vi "Raft_wars_Ver8.vi"() -> ()   [LabVIEW 2026]
panel:
  in  "Play Again":bool
  out "Computer Board":dbl[][](array[numeric])
  out "Player  Board":dbl[][](array[numeric])
  in  "Player Ship Inputs":T1(array[cluster]) {"Y-Coordinate" min=0 max=7; "X-Coordinate" min=0 max=7}
  in  "Emergency Stop":bool
  out "Game Status":string
  out "Ships Placed":dbl
  out "Losses":dbl
  out "Computer Hits":dbl
  out "Wins":dbl
  out "Player Hits":dbl
  in  "Attack":bool
  in  "Place Ship":bool
  in  "Attack Y":dbl
  in  "Attack X":dbl
  in  "Ship Y":dbl
  in  "Ship X":dbl
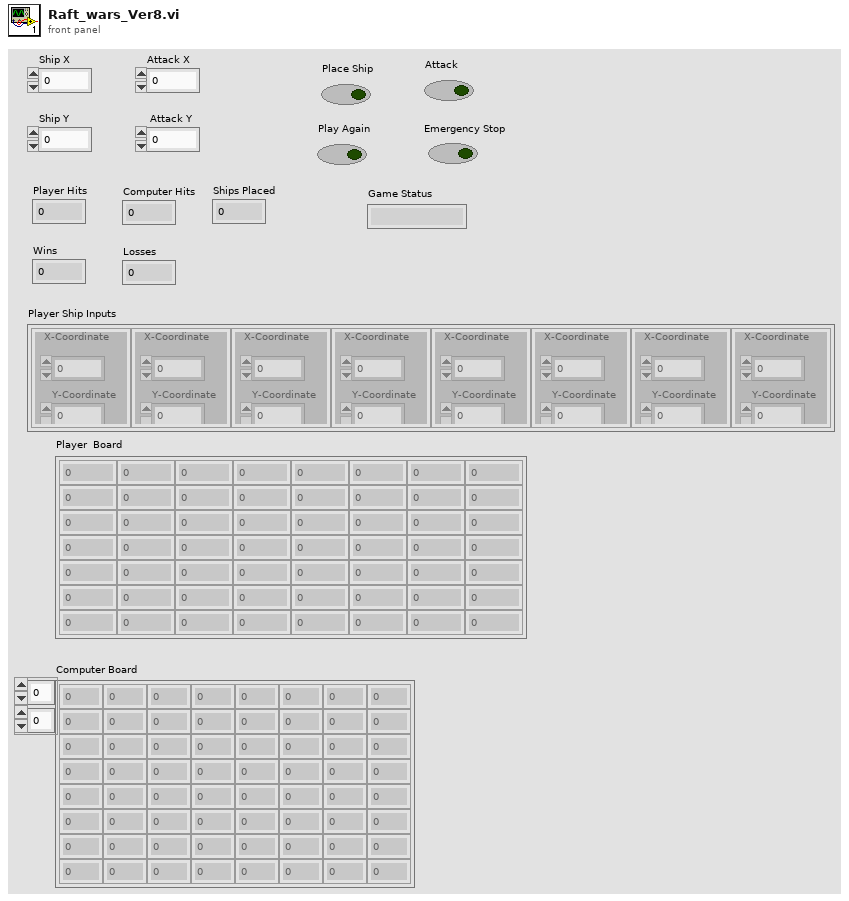
[diagram p1: front panel]
types:
  T1 = cluster{"X-Coordinate":i32, "Y-Coordinate":i32}[]
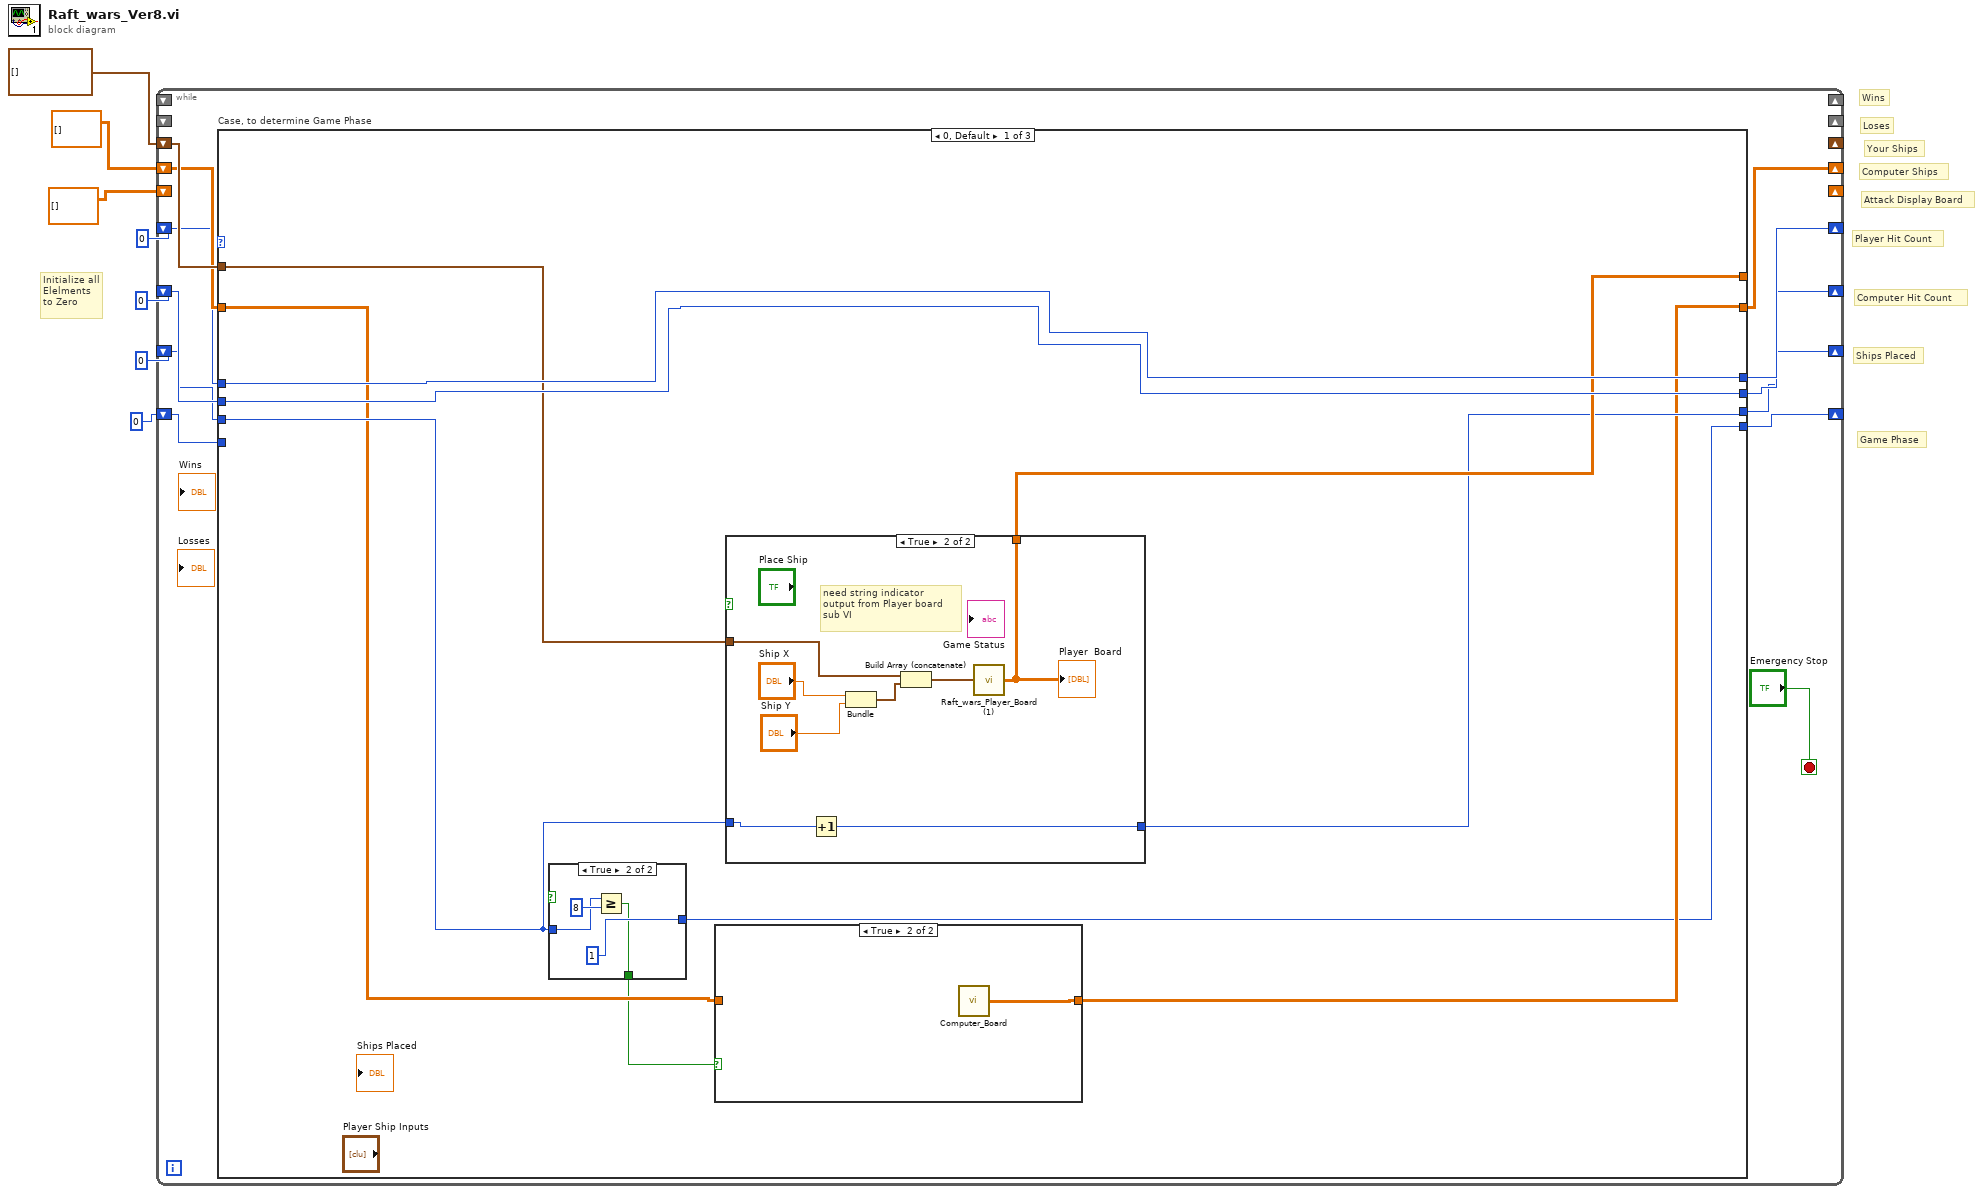
[diagram p0: block diagram]
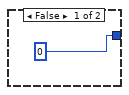
[diagram p3: hidden frame]
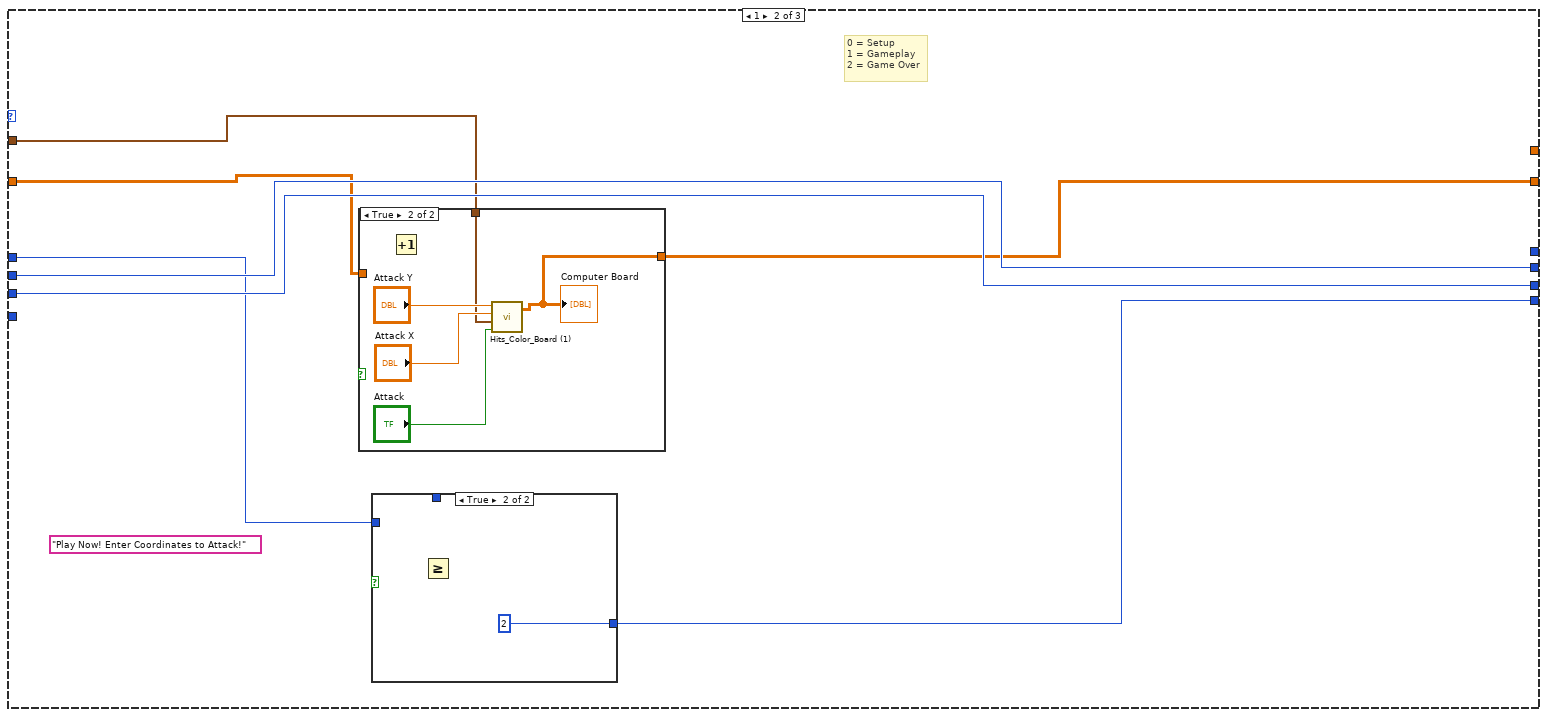
[diagram p5: hidden frame]
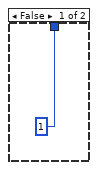
[diagram p6: hidden frame]
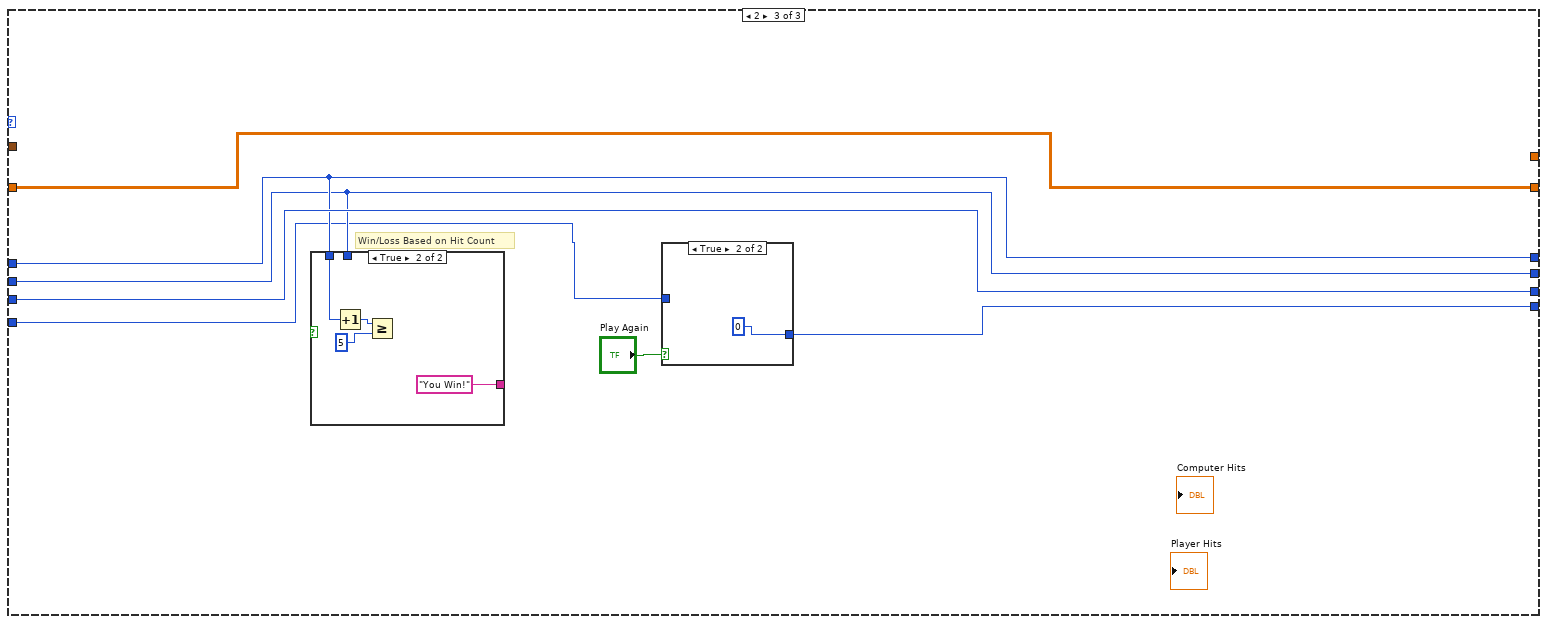
[diagram p8: hidden frame]
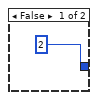
[diagram p9: hidden frame]
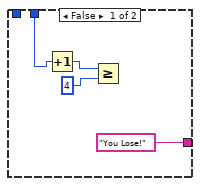
[diagram p10: hidden frame]
diagram:
  # "Loses"
  # "Wins"
  # "Attack Display Board"
  # "Initialize all\nElelments\nto Zero"
  # "Ships Placed"
  # "Your Ships"
  # "Computer Ships"
  # "Player Hit Count"
  # "Computer Hit Count"
  # "Game Phase"
  n1 = while {
    shift-right: _ -> [_]
    shift-left: cluster{i32, i32}[] [] -> [w18]
    shift-right: [w9] -> _
    shift-left: dbl[][] [] ("Array") -> [w17]
    shift-right: [w13] -> _
    shift-left: 0 -> [w16]
    shift-right: [w12] -> _
    shift-left: 0 -> [w15]
    shift-right: [w11] -> _
    shift-left: 0 -> [w14]
    shift-right: [w10] -> _
    shift-left: 0 -> [w8]
    shift-right: _ -> [_]
    shift-left: dbl[][] [] ("Array") -> [_]
    shift-right: _ -> [_]
    shift-left: _ -> [_]
    shift-right: _ -> [_]
    shift-left: _ -> [_]
    stop <- "Emergency Stop" stop-if-true
    n2 = case "Case, to determine Game Phase" shown="0, Default" {
      selector: _ -> [_ _ _]
      tunnel: w18 -> [w27 w46 _]
      tunnel: [w25 _ _] -> _
      tunnel: w17 -> [w21 w48 w66]
      tunnel: [w23 w49 w66] -> w9
      tunnel: w16 -> [w29 w47 w64]
      tunnel: w15 -> [w28 w51 w63]
      tunnel: w14 -> [w26 w52 w65]
      tunnel: [w29 _ w64] -> w13
      tunnel: [w28 w51 w63] -> w12
      tunnel: [w24 w52 w65] -> w11
      tunnel: [w22 w50 w62] -> w10
      tunnel: w8 -> [_ _ w60]
      frame 0, Default {
        n3 = case shown="True" {
          selector: _ -> [_ _]
          tunnel: w26 -> [_ w35]
          tunnel: [0 1] -> w22
          tunnel: [_ w33] -> w20
          frame False {
          }
          frame True {
            n4 = Greater Or Equal?(x=w35, y=8) -> (x >= y?=w33:bool)
          }
        }
        n5 = case shown="True" w20 {
          tunnel: w21 -> [w30 _]
          tunnel: [w30 w31] -> w23
          frame False {
          }
          frame True {
            n6 = call "Computer_Board.vi"() -> ("Array"=w31:dbl[][])
          }
        }
        n7 = case shown="True" {
          selector: _ -> [_ _]
          tunnel: w27 -> [_ w41]
          tunnel: w26 -> [w37 w39]
          tunnel: [_ w40] -> w25
          tunnel: [w37 w38] -> w24
          frame False {
          }
          frame True {
            # "need string indicator\noutput from Player board \nsub VI"
            n8 = Increment(x=w39) -> (x+1=w38:i32)
            n9 = Bundle("Ship X"="Ship X", "Ship Y"="Ship Y") -> (w43:cluster{"Ship X":dbl, "Ship Y":dbl})  [unwired: 1 in]
            n10 = Build Array (concatenate)(w41, w43) -> (w42:cluster{"Ship X":dbl, "Ship Y":dbl}[])
            n11 = call "Raft_wars_Player_Board (1).vi"("Player Ship Inputs"=w42) -> ("Array"=w40:dbl[][])
            "Player  Board" <- w40
          }
        }
      }
      frame 1 {
        (unwired) "Play Now! Enter Coordinates to Attack!"
        # "0 = Setup\n1 = Gameplay\n2 = Game Over"
        n12 = case shown="True" {
          selector: _ -> [_ _]
          tunnel: [_ w57] -> w49
          tunnel: w48 -> [_ _]
          tunnel: w46 -> [_ w55]
          frame False {
          }
          frame True {
            n13 = Increment() -> ()  [unwired: 1 in, 1 out]
            n14 = call "Hits_Color_Board (1).vi"("Attack Button"="Attack", "Player Ship Inputs"=w55, "X (col)"="Attack X", "Y (row)"="Attack Y") -> ("Attack Board"=w57:dbl[][])  [unwired: 1 out]
            "Computer Board" <- w57
          }
        }
        n15 = case shown="True" {
          selector: _ -> [_ _]
          tunnel: [_ 2] -> w50
          tunnel: [1 _] -> _
          tunnel: w47 -> [_ _]
          frame False {
          }
          frame True {
            n16 = Greater Or Equal?() -> ()  [unwired: 2 in, 1 out]
          }
        }
      }
      frame 2 {
        # "Win/Loss Based on Hit Count"
        n17 = case shown="True" {
          selector: _ -> [_ _]
          tunnel: w64 -> [_ w74]
          tunnel: ["You Lose!" "You Win!"] -> _
          tunnel: w63 -> [w70 _]
          frame False {
            n18 = Increment(x=w70) -> (x+1=w69:i32)
            n19 = Greater Or Equal?(x=w69, y=4) -> ()  [unwired: 1 out]
          }
          frame True {
            n20 = Increment(x=w74) -> (x+1=w73:i32)
            n21 = Greater Or Equal?(x=w73, y=5) -> ()  [unwired: 1 out]
          }
        }
        n22 = case shown="True" "Play Again" {
          tunnel: [2 0] -> w62
          tunnel: w60 -> [_ _]
          frame False {
          }
          frame True {
          }
        }
      }
    }
  }
